vi "GDSLvClass_AddMethod.vi"(0 "Class Refnum In":refnum<vi>, 1 "VI-Path":path, 5 "error in (no error)":errorcluster) -> (14 "Class Refnum Out":refnum<vi>, 15 "Add File":refnum<vi>, 19 "error out":errorcluster)   [LabVIEW 2016]
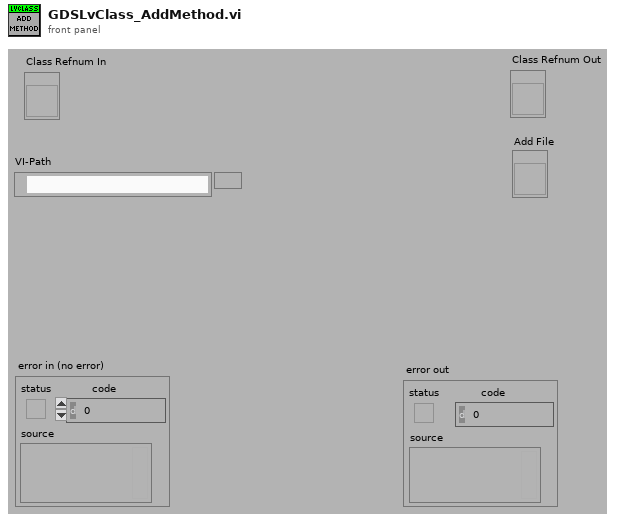
[diagram p1: front panel]
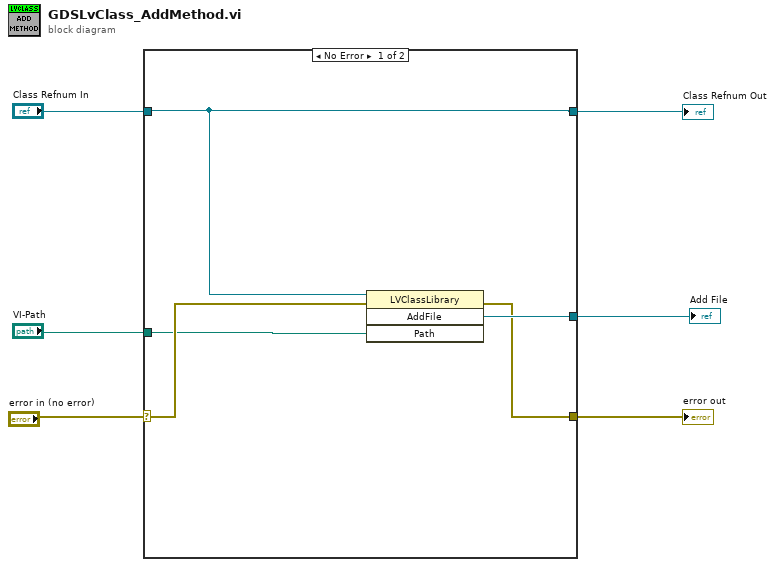
[diagram p0: block diagram]
diagram:
  n1 = case shown="No Error" "error in (no error)" {
    selector: "error in (no error)" -> [w11 w13]
    tunnel: [w8 w13] -> w5
    tunnel: "Class Refnum In" -> [w7 w12]
    tunnel: [w7 w12] -> w3
    tunnel: "VI-Path" -> [w10 _]
    tunnel: [w9 _] -> w1
    frame No Error {
      n2 = invoke class="LVClassLibrary" method="AddFile"(reference=w7, error in=w11, "Path"=w10) -> (error out=w8:errorcluster, "AddFile"=w9:refnum<vi>)  [unwired: 1 in, 2 out]
    }
    frame Error {
    }
  }
  "Class Refnum Out" <- w3
  "error out" <- w5
  "Add File" <- w1
